vi "SR_Thermal.vi"(11 "State Sample":refnum<class "RDS State.lvclass">) -> (1 "Thermal":T1, 2 "Thermal Points":sgl[](array[numeric]), 3 "State Sample Out":refnum<class "RDS State.lvclass">)   [LabVIEW 2015, in "Shore Library.lvlib"]
uses:
  Shore Library.lvlib
  RDS State Tracker/RDS State/RDS State.lvclass
  SR_Thermal.ctl
  RDS State Tracker/RDS State/RDS State.lvclass/RDS State.ctl
panel:
  # "PORT"
  # "FWD"
  # "AFT"
  # "STBD"
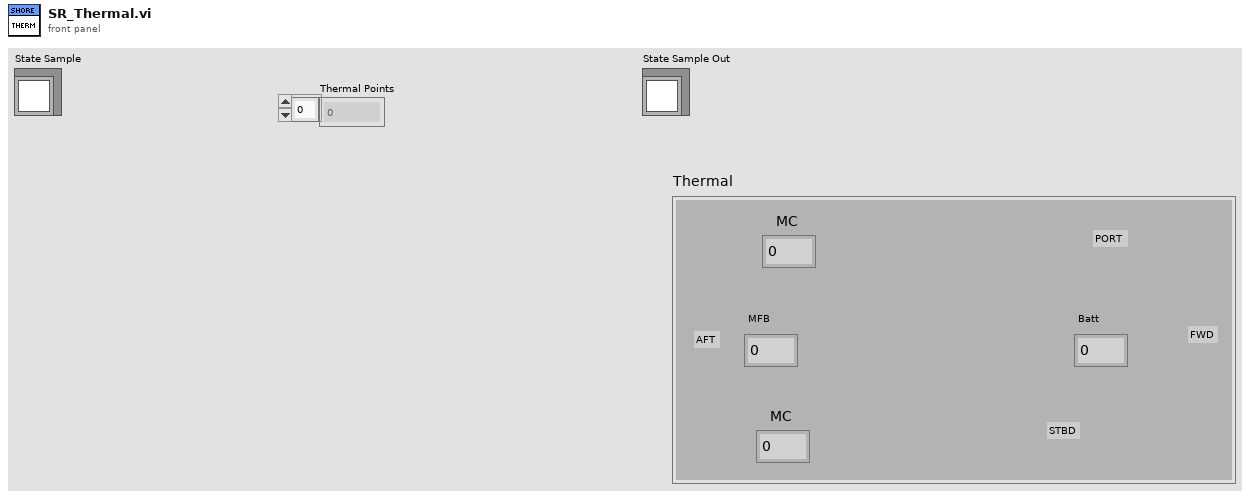
[diagram p1: front panel]
types:
  T1 = typedef "Shore Library.lvlib/SR_Thermal.ctl" = cluster{"Port MC":sgl, "Stbd MC":sgl, "Batt":sgl, "MFB":sgl}
  T2 = typedef "RDS Instrument Library.lvlib/Battery Data.ctl" = cluster{"Battery Status":T3, "Pack Voltage":sgl, "Pack Current":sgl, "Pack Capacity":sgl, "Max Cell Temp":sgl, "Min Cell Temp":sgl, "Max Cell Voltage":sgl, "Min Cell Voltage":sgl}
  T3 = typedef "RDS Instrument Library.lvlib/Battery Status.ctl" = enum16{"Pack Normal", "Alarm: Cell temp too high", "Alarm: Pack voltage too high", "Warn: Pack voltage too high ", "Alarm: Pack voltage too low", "Warn: Pack voltage low", "Alarm Pack current too high", "Warn: Pack current too high ", "Fault: Pack to chassis connection detected", "Fault: Pack to cell connection error", "Fautl: System error"}
  T4 = typedef "RDS Child Messages.lvlib/MCB Motor Status.ctl" = cluster{"Motor Power":i16, "Motor Command":i16, "Battery Volts":sgl, "Battery Amps":sgl, "Motor Amps":sgl, "MCU Temp":i16, "Heatsink Temp":i16, "Fault Flags":u16, "StatusFlags":u16}
  T5 = typedef "RDS Instrument Library.lvlib/Compass Data.ctl" = cluster{"Compass Heading":sgl, "pitch Angle":sgl, "roll Angle":sgl, "Temperature":sgl, "Depth":sgl, "Magnetic Field":sgl, "Magnetic Field X":sgl, "Magnetic Field Y":sgl, "Magnetic Field Z":sgl, "Acceleration":sgl, "Acceleration X":sgl, "Acceleration Y":sgl, "Gyro":sgl, "Gyro X":sgl, "Acceleration Z":sgl, "Gyro Y":sgl, "Raw Heading":sgl}
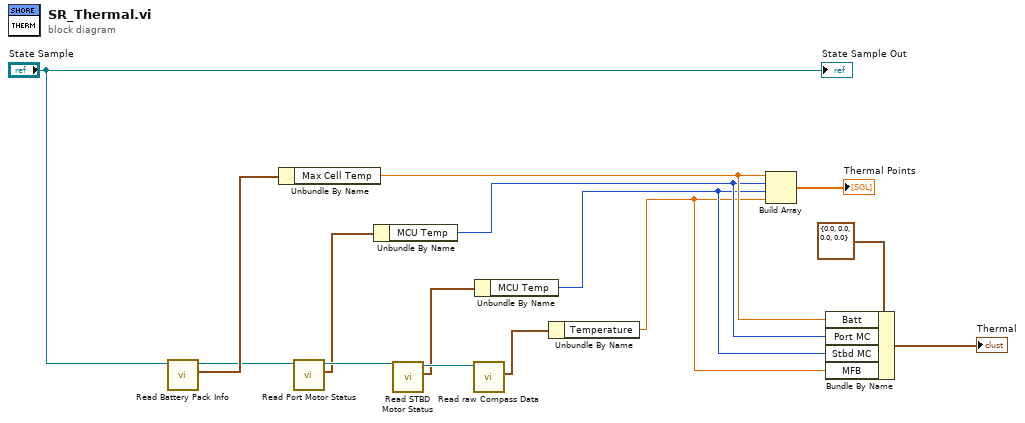
[diagram p0: block diagram]
diagram:
  n1 = call "Read Battery Pack Info.vi"("RDS State in"="State Sample") -> ("Battery Pack Info"=w14:T2, "RDS State out"=w13:refnum<class "RDS State.lvclass">)  [unwired: 8 in, 1 out]
  n2 = Unbundle By Name(w14) -> ("Max Cell Temp"=w4:sgl)
  n3 = call "Read Port Motor Status.vi"("RDS State in"=w13) -> ("Port Motor Data"=w10:T4, "RDS State out"=w12:refnum<class "RDS State.lvclass">)  [unwired: 8 in, 1 out]
  n4 = Unbundle By Name(w10) -> ("MCU Temp"=w3:i16)
  n5 = call "Read STBD Motor Status.vi"("RDS State in"=w12) -> ("STBD Motor"=w9:T4, "RDS State out"=w11:refnum<class "RDS State.lvclass">)  [unwired: 8 in, 1 out]
  n6 = call "Read raw Compass Data.vi"("RDS State in"=w11) -> ("Compass Data"=w8:T5)  [unwired: 8 in, 2 out]
  n7 = Unbundle By Name(w9) -> ("MCU Temp"=w2:i16)
  n8 = Unbundle By Name(w8) -> ("Temperature"=w1:sgl)
  n9 = Build Array(w4, w3, w2, w1) -> (→"Thermal Points":sgl[])
  n10 = Bundle By Name(cluster=T1 {"Port MC"=0.0, "Stbd MC"=0.0, "Batt"=0.0, "MFB"=0.0} ("Thermal 2"), "Batt"=w4, "Port MC"=w3, "Stbd MC"=w2, "MFB"=w1) -> (→"Thermal":T1)
  "State Sample Out" <- "State Sample"
